vi "Flatten JSON Object to JSONpath Array.vi"(4 "Maximum Depth":i32=-1, 6 "Initial Path":string="$", 7 "Include $Paths to Objects":bool, 8 "error in (no error)":errorcluster, 10 "Offset":i32, 11 "JSON":string) -> (0 "error out":errorcluster, 1 "<JSON>":string[](array[string]) caption="<JSON>Items", 3 "$Paths":string[](array[string]))   [LabVIEW 2020, in "JSONtext.lvlib"]
doc: "Takes a JSON Value and \"flattens\" the Object structure, producing out arrays of the $Paths to each item and the corresponding items. This works recursively on all subObjects (but not Arrays, which are treated as a single item).\n\nNote: to support names containing periods (.) in them, those names will be returned as a JSON string (quoted). \n\nFor example: the JSON {\"A\":{\"B1\":1,\"B2\":\"x\"},\"A2\":true,\"A.1\":{\"C\":123}} produces the arrays:\n$Paths (Items):\n$.A.B1 (1)\n$.A.B2 (\"x\")\n$.A2 (true)\n$.\"A.1\".C (123)\n\nIf \"Include $Paths to Objects\" is True, then the above list will incude a path to all Objects (including the root Object path \"$\"):\n$\n$.A\n$.A.B1\n$.A.B2\n$.A2\n$.\"A.1\"\n$.\"A.1\".C"
uses:
  <vilib>/JDP Science/JSONtext/JSONtext.lvlib
  <vilib>/JDP Science/JSONtext/support/quote and escape json string 2.vi
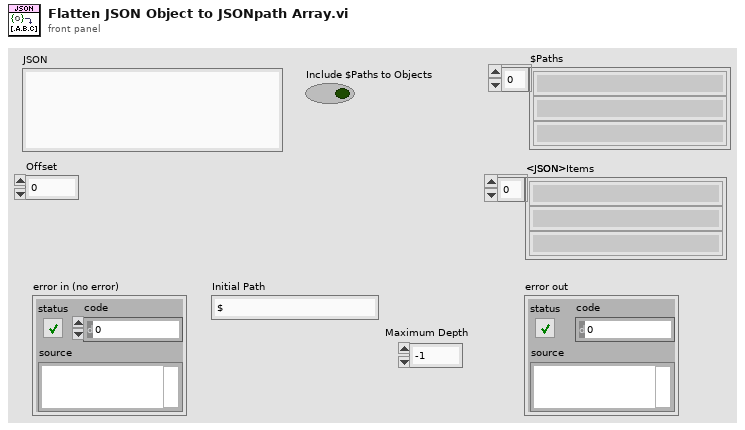
[diagram p1: front panel]
types:
  T1 = typedef "JSONtext.lvlib/JSON Value Type.ctl" = enum16{"Not a JSON Value", "JSON Object", "JSON Array", "String", "Number", "true", "false", "null"}
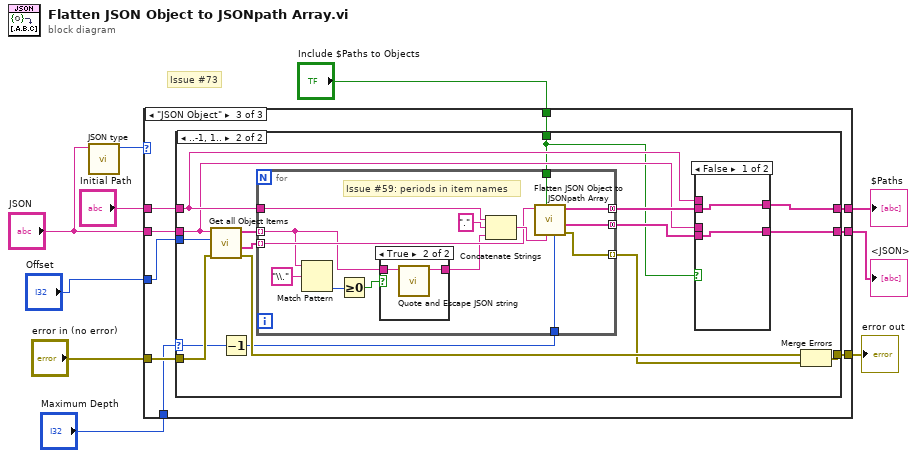
[diagram p0: block diagram]
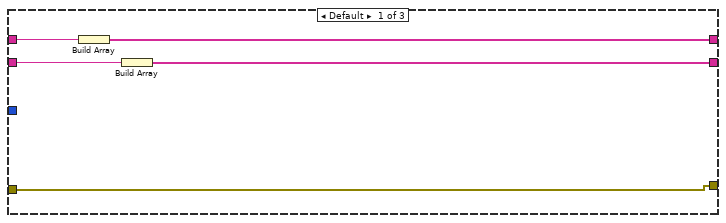
[diagram p2: hidden frame]
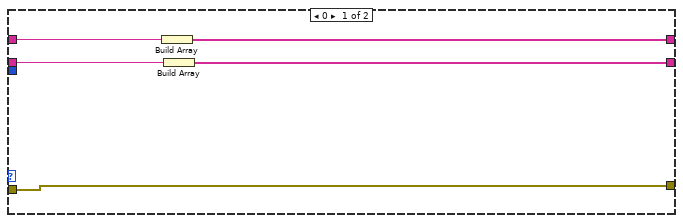
[diagram p4: hidden frame]
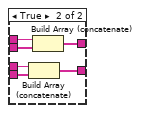
[diagram p5: hidden frame]
diagram:
  # "Issue #73"
  n1 = call <vilib>:"JSON type.vi"("JSON"="JSON") -> ("JSON Value Type"=w6:T1)  [unwired: 9 in, 1 out]
  n2 = case shown="\"JSON Object\"" w6 {
    tunnel: "JSON" -> [w15 _ w25]
    tunnel: [w12 _ w23] -> w7
    tunnel: [w14 _ w22] -> w8
    tunnel: "Initial Path" -> [w13 _ w24]
    tunnel: "Offset" -> [_ _ w21]
    tunnel: "error in (no error)" -> [w11 w16 w20]
    tunnel: [w11 w16 w19] -> w3
    tunnel: "Maximum Depth" -> [_ _ w18]
    tunnel: "Include $Paths to Objects" -> [_ _ w17]
    frame Default {
      n3 = Build Array(w13) -> (w12:string[])
      n4 = Build Array(w15) -> (w14:string[])
    }
    frame "Not a JSON Value" {
    }
    frame "JSON Object" {
      n5 = case shown="..-1, 1.." w18 {
        selector: w18 -> [_ w37]
        tunnel: w25 -> [w28 w32]
        tunnel: w24 -> [w30 w34]
        tunnel: [w29 w35] -> w23
        tunnel: [w27 w33] -> w22
        tunnel: w21 -> [_ w42]
        tunnel: w20 -> [w26 w41]
        tunnel: [w26 w39] -> w19
        tunnel: w17 -> [_ w31]
        frame 0 {
          n6 = Build Array(w30) -> (w29:string[])
          n7 = Build Array(w28) -> (w27:string[])
        }
        frame ..-1, 1.. {
          n8 = call <vilib>:"Get all Object Items.vi"("error in (no error)"=w41, "Offset"=w42, "JSON"=w32) -> ("error out"=w40:errorcluster, "<JSON>"=w44:string[], "Item Names"=w45:string[])  [unwired: 5 in, 1 out]
          n9 = Decrement(x=w37) -> (x-1=w36:i32)
          n10 = for {
            tunnel: w34 -> [w68]
            tunnel: [w66] -> w46 mode=concatenating
            tunnel: w45 -> [w59] mode=indexing
            tunnel: w44 -> [w64] mode=indexing
            tunnel: [w63] -> w43 mode=concatenating
            tunnel: [w62] -> w38 mode=indexing
            tunnel: w36 -> [w56]
            tunnel: w31 -> [w55]
            # "Issue #59: periods in item names"
            n11 = Match Pattern(string=w59, regular expression="\\.") -> (offset past match=w60:i32)  [unwired: 1 in, 3 out]
            n12 = Greater Or Equal To 0?(x=w60) -> (x >= 0?=w57:bool)
            n13 = case shown="True" w57 {
              tunnel: w59 -> [w69 w71]
              tunnel: [w69 w70] -> w58
              frame False {
              }
              frame True {
                n14 = call <vilib>:"Quote and Escape JSON string.vi"("Plain Text"=w71) -> ("<JSON>"=w70:string)  [unwired: 10 in]
              }
            }
            n15 = Concatenate Strings(w68, "." ("string"), w58) -> (w65:string)
            n16 = call <vilib>:"Flatten JSON Object to JSONpath Array.vi"("Maximum Depth"=w56, "Initial Path"=w65, "Include $Paths to Objects"=w55, "JSON"=w64) -> ("error out"=w62:errorcluster, "<JSON>"=w63:string[], "$Paths"=w66:string[])  [unwired: 5 in]
          }
          n17 = case shown="False" w31 {
            tunnel: w46 -> [w48 w54]
            tunnel: w43 -> [w47 w53]
            tunnel: [w48 w52] -> w35
            tunnel: w34 -> [_ w51]
            tunnel: [w47 w50] -> w33
            tunnel: w32 -> [_ w49]
            frame False {
            }
            frame True {
              n18 = Build Array (concatenate)(w49, w53) -> (w50:string[])
              n19 = Build Array (concatenate)(w51, w54) -> (w52:string[])
            }
          }
          n20 = Merge Errors(w40, w38) -> (w39:errorcluster)
        }
      }
    }
  }
  "<JSON>" <- w8
  "$Paths" <- w7
  "error out" <- w3
